vi "UploadToTarget.vi"(8 "error in (no error)":errorcluster, 9 "previousName":string, 10 "ConnectionData":T2, 11 "ConfigXMLControls":T1) -> (0 "error out":errorcluster, 3 "newName":string)   [LabVIEW 2015]
uses:
  General/RemoteFiles/connectionData.ctl
  ConfigXMLControl.ctl
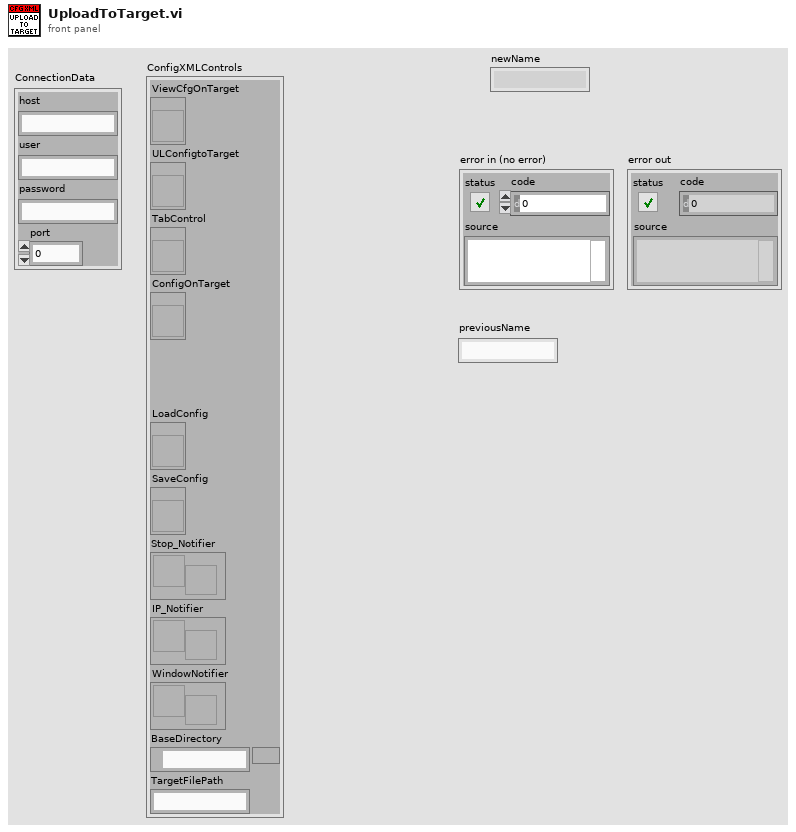
[diagram p1: front panel]
types:
  T1 = typedef "ConfigXMLControl.ctl" = cluster{"ViewCfgOnTarget":refnum<vi>, "ULConfigtoTarget":refnum<vi>, "TabControl":refnum<vi>, "ConfigOnTarget":refnum<vi>, "LoadConfig":refnum<vi>, "SaveConfig":refnum<vi>, "Stop_Notifier":refnum<notifier>, "IP_Notifier":refnum<notifier>, "WindowNotifier":refnum<notifier>, "BaseDirectory":path, "TargetFilePath":string}
  T2 = typedef "connectionData.ctl" = cluster{"host":string, "user":string, "password":string, "port":u16}
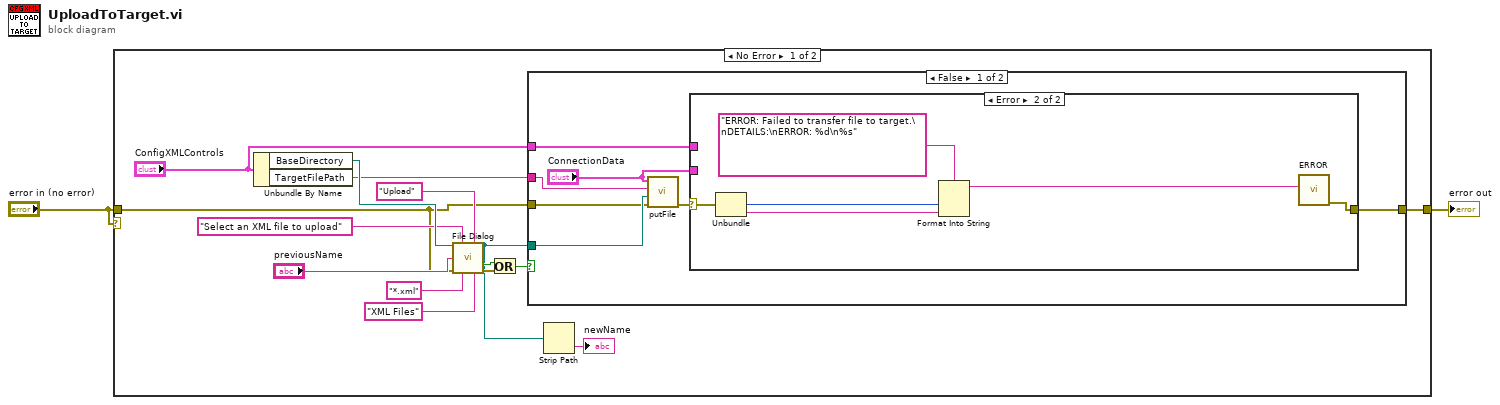
[diagram p0: block diagram]
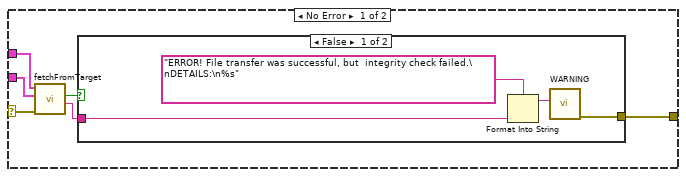
[diagram p2: hidden frame]
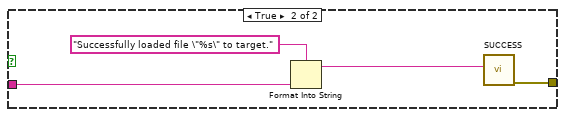
[diagram p3: hidden frame]
diagram:
  n1 = case shown="No Error" "error in (no error)" {
    tunnel: "error in (no error)" -> [w7 w46]
    tunnel: [w5 w46] -> w1
    frame No Error {
      n2 = Unbundle By Name("ConfigXMLControls") -> ("BaseDirectory"=w14:path, "TargetFilePath"=w8:string)
      n3 = call "File Dialog"("start path"=w14, "prompt"="Select an XML file to upload", "button label"="Upload", "default name"="previousName", "error in"=w7, "pattern (all files)"="*.xml", "pattern label"="XML Files") -> ("selected path"=w4:path, "cancelled"=w11:bool, "error out"=w10:errorcluster)  [unwired: 5 in, 1 out]
      n4 = Or(x=w11, y=w10) -> (x .or. y?=w9:bool)
      n5 = case shown="False" w9 {
        tunnel: w4 -> [w23 _]
        tunnel: w8 -> [w24 _]
        tunnel: w7 -> [w22 w45]
        tunnel: "ConfigXMLControls" -> [w19 _]
        tunnel: [w18 w45] -> w5
        frame False {
          n6 = call "putFile.vi"("error in (no error)"=w22, "local path"=w23, "remote path"=w24, "ConnectionData"="ConnectionData") -> ("error out"=w21:errorcluster)  [unwired: 6 in, 1 out]
          n7 = case shown="Error" w21 {
            selector: w21 -> [w28 w43]
            tunnel: "ConnectionData" -> [w30 _]
            tunnel: w19 -> [w29 _]
            tunnel: [w25 w39] -> w18
            frame No Error {
              n8 = call "fetchFromTarget.vi"("error in (no error)"=w28, "ConnectionData"=w30, "ConfigXMLControls"=w29) -> ("nameMessageOut"=w26:string, "SuccessfulRead?"=w27:bool)  [unwired: 5 in, 2 out]
              n9 = case shown="False" w27 {
                tunnel: w26 -> [w33 w37]
                tunnel: [w31 w35] -> w25
                frame False {
                  n10 = Format Into String(format string="ERROR! File transfer was successful, but  integrity check failed.\nDETAILS:\n%s" ("Message"), w33) -> (resulting string=w32:string)  [unwired: 2 in, 1 out]
                  n11 = call "WARNING"("Message"=w32) -> ("error out"=w31:errorcluster)  [unwired: 9 in, 1 out]
                }
                frame True {
                  n12 = Format Into String(format string="Successfully loaded file \"%s\" to target." ("Message"), w37) -> (resulting string=w36:string)  [unwired: 2 in, 1 out]
                  n13 = call "SUCCESS"("Message"=w36) -> ("error out"=w35:errorcluster)  [unwired: 9 in, 1 out]
                }
              }
            }
            frame Error {
              n14 = Unbundle(w43) -> ("code"=w42:i32, "source"=w41:string)  [unwired: 1 out]
              n15 = Format Into String(format string="ERROR: Failed to transfer file to target.\nDETAILS:\nERROR: %d\n%s", w42, w41) -> (resulting string=w40:string)  [unwired: 2 in, 1 out]
              n16 = call "ERROR"("Message"=w40) -> ("error out"=w39:errorcluster)  [unwired: 9 in, 1 out]
            }
          }
        }
        frame True {
          # "If true, do not upload"
        }
      }
      n17 = Strip Path(path=w4) -> (name=→"newName":string)  [unwired: 1 out]
    }
    frame Error {
    }
  }
  "error out" <- w1
